vi "Set cif_management_common_PluginStatusData.vi"(7 "Complete Call (T)":bool=TRUE, 8 "error in (no error)":errorcluster, 10 "package_templatemessage":T1, 11 "gRPCid":T10) -> (0 "error out":errorcluster)   [LabVIEW 2021, in "CIFCoreChannel_server.lvlib"]
uses:
  CIFCoreChannel_server.lvlib
  <vilib>/gRPC/LabVIEW gRPC Library/Shared/grpcId.ctl
  cif_management_common_PluginStatusData.ctl
  cif_management_common_PluginStatusData_PluginState.ctl
  cif_management_common_TimingStatistics.ctl
  cif_common_TimingStats.ctl
  cif_management_common_FifoStatistics.ctl
  cif_management_common_Error.ctl
  cif_management_common_MonitorDoubles.ctl
  cif_management_common_MonitorU64.ctl
  cif_management_common_MonitorI64.ctl
  cif_management_common_PluginStatusData_Flat.ctl
  cif_management_common_TimingStatistics_Flat.ctl
  cif_common_TimingStats_Flat.ctl
  cif_management_common_FifoStatistics_Flat.ctl
  cif_management_common_Error_Flat.ctl
  cif_management_common_MonitorDoubles_Flat.ctl
  cif_management_common_MonitorU64_Flat.ctl
  cif_management_common_MonitorI64_Flat.ctl
  dcc74a39-081a-4bdd-860b-8ed792803c96.vi
  <vilib>/gRPC/LabVIEW gRPC Library/Shared/TranslateGrpcError.vi
  RichToFlatcif_management_common_TimingStatistics.vi
  RichToFlatcif_management_common_FifoStatistics.vi
  RichToFlatcif_management_common_Error.vi
  RichToFlatcif_management_common_MonitorDoubles.vi
  RichToFlatcif_management_common_MonitorU64.vi
  RichToFlatcif_management_common_MonitorI64.vi
  RichToFlatcif_common_TimingStats.vi
  <vilib>/gRPC/LabVIEW gRPC Library/Server API/Server/Get Server DLL Path.vi
  <vilib>/Utility/error.llb/Error Cluster From Error Code.vi
  <vilib>/gRPC/LabVIEW gRPC Library/grpc-lvsupport-release.lvlib
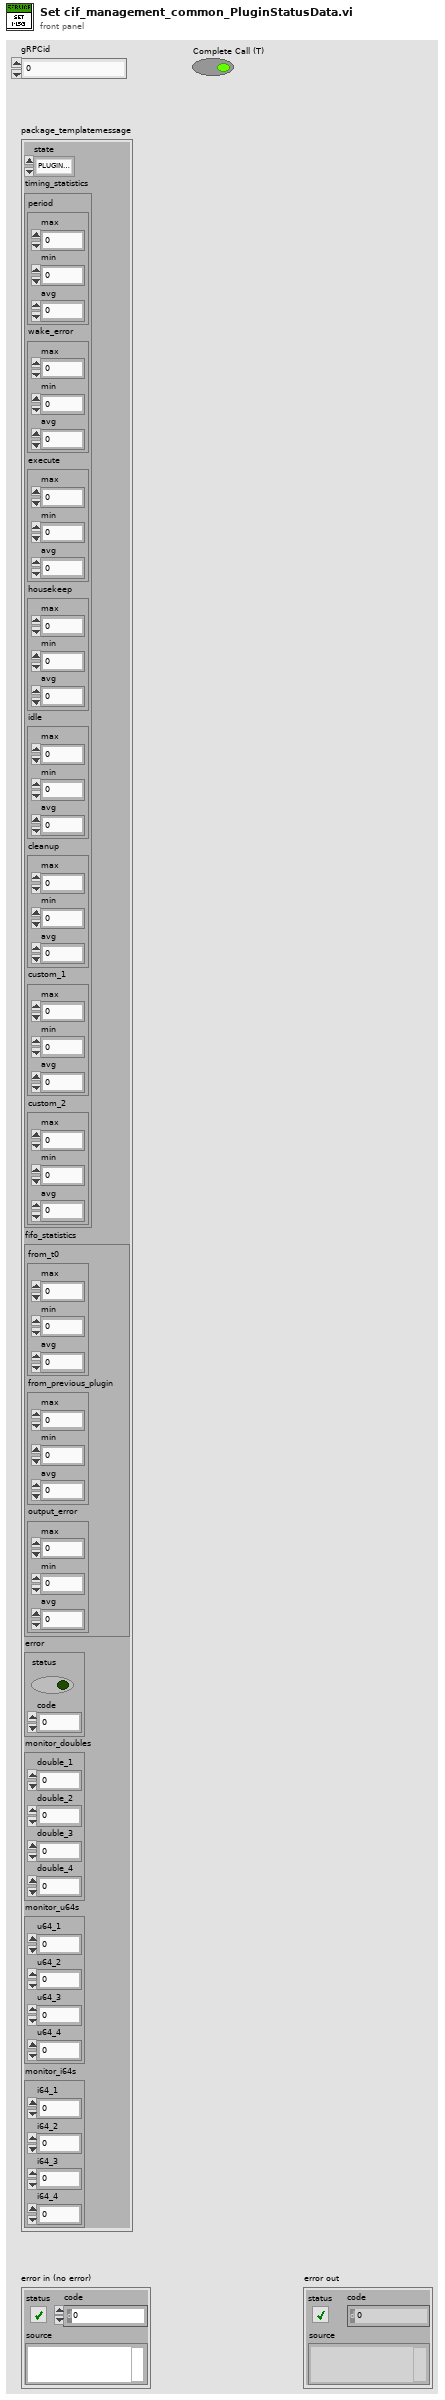
[diagram p1: front panel]
types:
  T1 = typedef "CIFCoreChannel_server.lvlib/cif_management_common_PluginStatusData.ctl" = cluster{"state":T2, "timing_statistics":T3, "fifo_statistics":T5, "error":T6, "monitor_doubles":T7, "monitor_u64s":T8, "monitor_i64s":T9}
  T2 = typedef "CIFCoreChannel_server.lvlib/cif_management_common_PluginStatusData_PluginState.ctl" = enum32{"PLUGINSTATE_UNKNOWN", "PLUGINSTATE_CREATING", "PLUGINSTATE_LISTENING", "PLUGINSTATE_RUNNING", "PLUGINSTATE_CLEANINGUP", "PLUGINSTATE_DESTROYING"}
  T3 = typedef "CIFCoreChannel_server.lvlib/cif_management_common_TimingStatistics.ctl" = cluster{"period":T4, "wake_error":T4, "execute":T4, "housekeep":T4, "idle":T4, "cleanup":T4, "custom_1":T4, "custom_2":T4}
  T4 = typedef "CIFCoreChannel_server.lvlib/cif_common_TimingStats.ctl" = cluster{"max":i64, "min":i64, "avg":dbl}
  T5 = typedef "CIFCoreChannel_server.lvlib/cif_management_common_FifoStatistics.ctl" = cluster{"from_t0":T4, "from_previous_plugin":T4, "output_error":T4}
  T6 = typedef "CIFCoreChannel_server.lvlib/cif_management_common_Error.ctl" = cluster{"status":bool, "code":i32}
  T7 = typedef "CIFCoreChannel_server.lvlib/cif_management_common_MonitorDoubles.ctl" = cluster{"double_1":dbl, "double_2":dbl, "double_3":dbl, "double_4":dbl}
  T8 = typedef "CIFCoreChannel_server.lvlib/cif_management_common_MonitorU64.ctl" = cluster{"u64_1":u64, "u64_2":u64, "u64_3":u64, "u64_4":u64}
  T9 = typedef "CIFCoreChannel_server.lvlib/cif_management_common_MonitorI64.ctl" = cluster{"i64_1":i64, "i64_2":i64, "i64_3":i64, "i64_4":i64}
  T10 = typedef "grpc-lvsupport-release.lvlib/grpcId.ctl" = u64
  T11 = typedef "CIFCoreChannel_server.lvlib/cif_management_common_PluginStatusData_Flat.ctl" = cluster{"state":T2, "timing_statistics":T12, "fifo_statistics":T14, "error":T15, "monitor_doubles":T16, "monitor_u64s":T17, "monitor_i64s":T18}
  T12 = typedef "CIFCoreChannel_server.lvlib/cif_management_common_TimingStatistics_Flat.ctl" = cluster{"period":T13, "wake_error":T13, "execute":T13, "housekeep":T13, "idle":T13, "cleanup":T13, "custom_1":T13, "custom_2":T13}
  T13 = typedef "CIFCoreChannel_server.lvlib/cif_common_TimingStats_Flat.ctl" = cluster{"max":i64, "min":i64, "avg":dbl}
  T14 = typedef "CIFCoreChannel_server.lvlib/cif_management_common_FifoStatistics_Flat.ctl" = cluster{"from_t0":T13, "from_previous_plugin":T13, "output_error":T13}
  T15 = typedef "CIFCoreChannel_server.lvlib/cif_management_common_Error_Flat.ctl" = cluster{"status":bool, "code":i32}
  T16 = typedef "CIFCoreChannel_server.lvlib/cif_management_common_MonitorDoubles_Flat.ctl" = cluster{"double_1":dbl, "double_2":dbl, "double_3":dbl, "double_4":dbl}
  T17 = typedef "CIFCoreChannel_server.lvlib/cif_management_common_MonitorU64_Flat.ctl" = cluster{"u64_1":u64, "u64_2":u64, "u64_3":u64, "u64_4":u64}
  T18 = typedef "CIFCoreChannel_server.lvlib/cif_management_common_MonitorI64_Flat.ctl" = cluster{"i64_1":i64, "i64_2":i64, "i64_3":i64, "i64_4":i64}
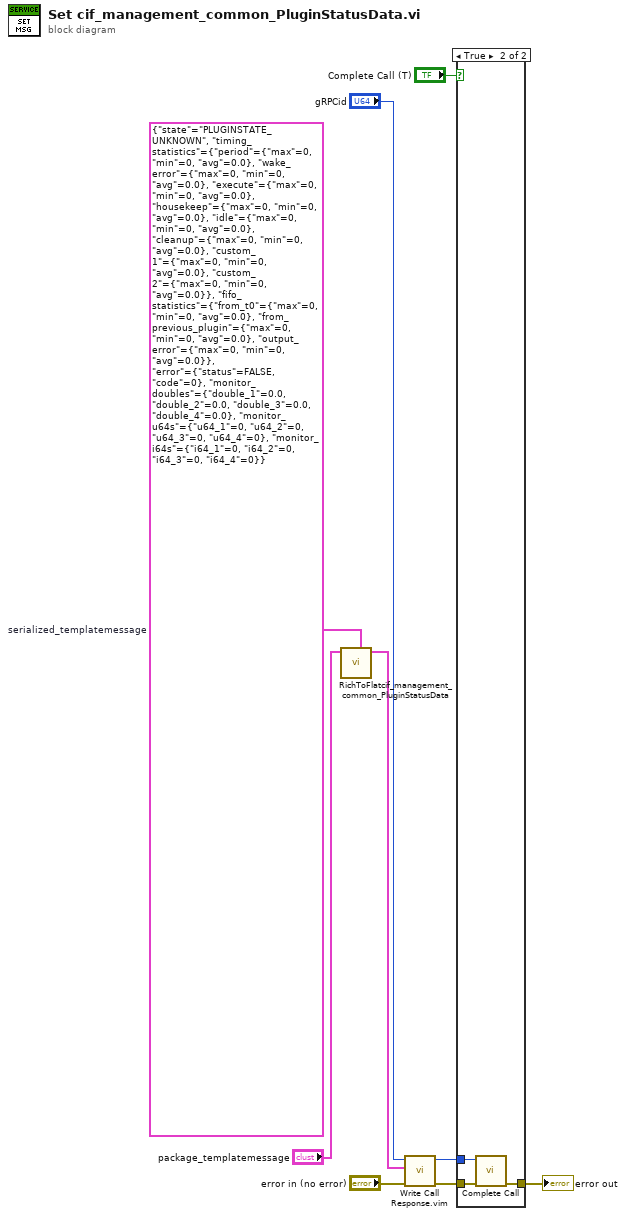
[diagram p0: block diagram]
diagram:
  w2 = T11 {"state"=enum."PLUGINSTATE_UNKNOWN", "timing_statistics"={"period"={"max"=0, "min"=0, "avg"=0.0}, "wake_error"={"max"=0, "min"=0, "avg"=0.0}, "execute"={"max"=0, "min"=0, "avg"=0.0}, "housekeep"={"max"=0, "min"=0, "avg"=0.0}, "idle"={"max"=0, "min"=0, "avg"=0.0}, "cleanup"={"max"=0, "min"=0, "avg"=0.0}, "custom_1"={"max"=0, "min"=0, "avg"=0.0}, "custom_2"={"max"=0, "min"=0, "avg"=0.0}}, "fifo_statistics"={"from_t0"={"max"=0, "min"=0, "avg"=0.0}, "from_previous_plugin"={"max"=0, "min"=0, "avg"=0.0}, "output_error"={"max"=0, "min"=0, "avg"=0.0}}, "error"={"status"=FALSE, "code"=0}, "monitor_doubles"={"double_1"=0.0, "double_2"=0.0, "double_3"=0.0, "double_4"=0.0}, "monitor_u64s"={"u64_1"=0, "u64_2"=0, "u64_3"=0, "u64_4"=0}, "monitor_i64s"={"i64_1"=0, "i64_2"=0, "i64_3"=0, "i64_4"=0}}  # serialized_templatemessage
  n1 = call "RichToFlatcif_management_common_PluginStatusData.vi"("OutputClusterType"=w2, "InputCluster"="package_templatemessage") -> ("OutputCluster"=w1:T11)  [unwired: 9 in]
  n2 = call "Write Call Response.vim"("error in"="error in (no error)", "Response Data"=w1, "gRPCid in"="gRPCid") -> ("error out"=w6:errorcluster, "gRPCid out"=w7:T10)  [unwired: 7 in]
  n3 = case shown="True" "Complete Call (T)" {
    tunnel: [w10 w13] -> w9
    tunnel: w7 -> [_ w12]
    tunnel: w6 -> [w10 w11]
    frame False {
    }
    frame True {
      n4 = call <vilib>:"Complete Call.vi"("gRPCid"=w12, "error in"=w11) -> ("error out"=w13:errorcluster)  [unwired: 8 in]
    }
  }
  "error out" <- w9
